vi "InitializeFile.vi"(8 "error in (no error)":errorcluster caption="错误输入（无错误）", 11 "XML File Path":path=path "C:/Users/user/Desktop/1.xml") -> (2 "大小":i32, 3 "Point":T1[](array[typedef]))   [LabVIEW 2017]
uses:
  Ctrls/Point.ctl
  <vilib>/Utility/xml.llb/Read From XML File(string).vi
panel:
  out "error out":errorcluster caption="错误输出"
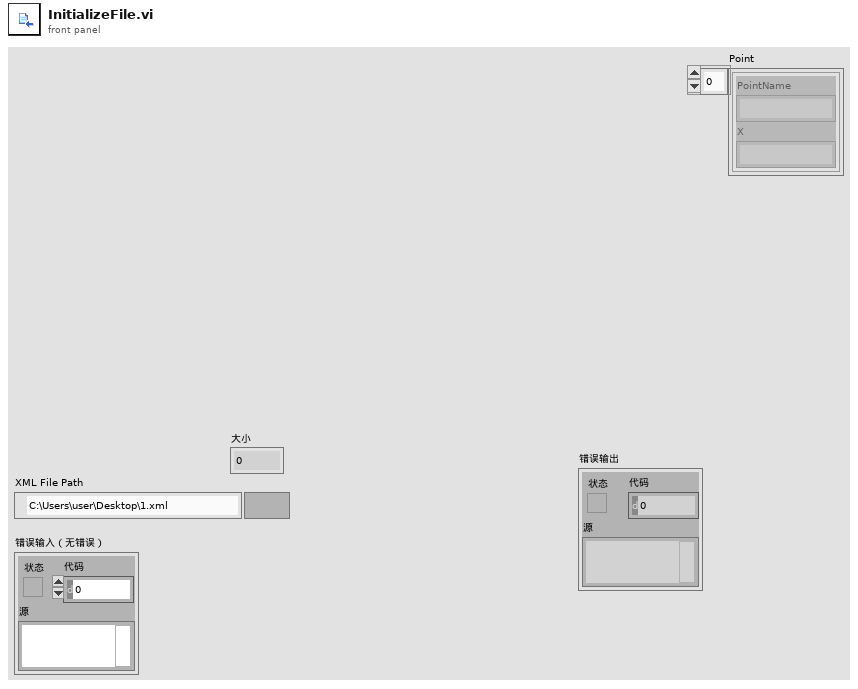
[diagram p1: front panel]
types:
  T1 = typedef "Point.ctl" = cluster{"PointName":string, "X":string}
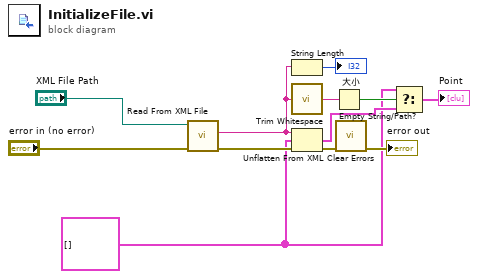
[diagram p0: block diagram]
diagram:
  w2 = T1[] [] ("t")
  n1 = call-poly <vilib>:"Read From XML File.vi"("error in (no error)"="error in (no error)", "XML File Path"="XML File Path") -> ("error out"=w10:errorcluster, "XML Elements"=w3:string)  [unwired: 7 in, 1 out]
  n2 = String Length(string=w3) -> (length=→"大小":i32)
  n3 = call <vilib>:"Trim Whitespace.vi"("string"=w3) -> ("trimmed string"=w6:string)  [unwired: 1 in]
  n4 = Unflatten From XML(xml string=w3, type=w2, error in (no error)=w10) -> (value=w4:T1[], error out=w9:errorcluster)
  n5 = Empty String/Path?(string/path=w6) -> (empty?=w5:bool)
  n6 = call <vilib>:"Clear Errors.vi"("error in (no error)"=w9) -> ("error out"=→"error out":errorcluster)  [unwired: 5 in, 1 out]
  n7 = Select(t=w2, s=w5, f=w4) -> (s? t:f=→"Point":T1[])
